vi "_LogFirmwareEvents.vi"(0 "Event":string="117:52:56, Lost Communication - Check Ethernet Connection.\n117:52:56, Going to Lost Communication state.\n117:52:56, Instr State transitioned from Ready to Lost Communication; FPGA Running = FALSE; Run Mode = 1; Loop = 431971.\n117:52:56, Heater Power Supply Error; Instr State = Lost Communication.\n117:52:56, PC Communication Established\n117:55:43, Start Run: Instr State = Lost Communication; FPGA Running = FALSE;  Time Out = FALSE.\n117:55:44, Analyzer is Ready\n117:55:52, Start Run: Instr State = Ready; FPGA Running = FALSE;  Time Out = FALSE.\n117:55:56, Heater Power Supply Error; Instr State = Ready.") -> ()   [LabVIEW 2015]
doc: "This vi maintains a datalog file for plate positions in motor steps.\nEach datalog record consists of the following data members:\nData/time in secs from 12am 1/1/1904.\nHorizontal motor steps\nVertical motor steps\nAll numbers are stored as 8-byte doubles."
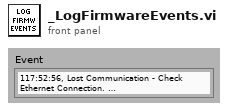
[diagram p1: front panel]
types:
  T1 = enum16{"open", "replace", "create", "open or create", "replace or create", "replace or create with confirmation"}
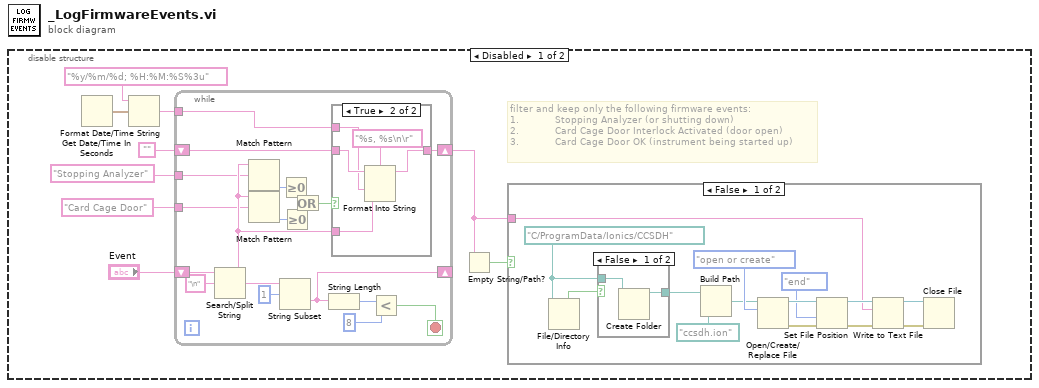
[diagram p0: block diagram]
diagram:
  n1 = disable-structure shown="Disabled" {
    frame Disabled {
      # "filter and keep only the following firmware events:\n1.            Stopping Analyzer (or shutting down)\n2.            Card Cage Door Interlock Activated (door open)\n3.            Card Cage Door OK (instrument being started up)"
      n2 = Get Date/Time In Seconds() -> (seconds since 1Jan1904=w6:timestamp)
      n3 = Format Date/Time String(time format string (%c)="%y/%m/%d; %H:%M:%S%3u", seconds (now)=w6) -> (date/time string=w4:string)  [unwired: 1 out]
      n4 = while {
        shift-right: [w19] -> w3
        shift-left: "" -> [w20]
        tunnel: w4 -> [w18]
        shift-right: [w24] -> _
        shift-left: "Event" -> [w28]
        tunnel: "Stopping Analyzer" -> [w16]
        tunnel: "Card Cage Door" -> [w15]
        stop <- w22 stop-if-true
        n5 = Search/Split String(string=w28, search string/char (-)="\n") -> (substring before match=w17:string, match + rest of string=w26:string)  [unwired: 1 in, 1 out]
        n6 = Match Pattern(string=w17, regular expression=w16) -> (offset past match=w14:i32)  [unwired: 1 in, 3 out]
        n7 = Match Pattern(string=w17, regular expression=w15) -> (offset past match=w13:i32)  [unwired: 1 in, 3 out]
        n8 = String Subset(string=w26, offset (0)=1) -> (substring=w24:string)  [unwired: 1 in]
        n9 = Greater Or Equal To 0?(x=w14) -> (x >= 0?=w11:bool)
        n10 = Greater Or Equal To 0?(x=w13) -> (x >= 0?=w10:bool)
        n11 = Or(x=w11, y=w10) -> (x .or. y?=w12:bool)
        n12 = String Length(string=w24) -> (length=w23:i32)
        n13 = case shown="True" w12 {
          tunnel: w20 -> [w29 w33]
          tunnel: [w29 w30] -> w19
          tunnel: w18 -> [_ w32]
          tunnel: w17 -> [_ w31]
          frame False {
          }
          frame True {
            n14 = Format Into String(format string="%s, %s\n\r" ("Format String"), initial string=w33, w32, w31) -> (resulting string=w30:string)  [unwired: 1 in, 1 out]
          }
        }
        n15 = Less?(x=w23, y=8) -> (x < y?=w22:bool)
      }
      n16 = Empty String/Path?(string/path=w3) -> (empty?=w9:bool)
      n17 = case shown="False" w9 {
        tunnel: w3 -> [w35 _]
        frame False {
          w47 = path "C:/ProgramData/Ionics/CCSDH" ("path")
          n18 = File/Directory Info(path=w47) -> (directory=w48:bool)  [unwired: 1 in, 6 out]
          n19 = case shown="False" w48 {
            tunnel: w47 -> [w50 w51]
            tunnel: [w49 w51] -> w46
            frame False {
              n20 = Create Folder(path (use dialog)=w50) -> (created path=w49:path)  [unwired: 2 in, 2 out]
            }
            frame True {
            }
          }
          n21 = Build Path(base path=w46, name or relative path=path "ccsdh.ion" ("configuration file path")) -> (appended path=w43:path)
          n22 = Open/Create/Replace File(file path (use dialog)=w43, operation (0:open)=T1."open or create") -> (refnum out=w40:refnum<file>, error out=w38:errorcluster)  [unwired: 4 in, 1 out]
          n23 = Set File Position(refnum=w40, from (0:start)=enum16{"start", "end", "current"}."end", error in=w38) -> (refnum out=w39:refnum<file>, error out=w37:errorcluster)  [unwired: 1 in]
          n24 = Write to Text File(file (use dialog)=w39, text=w35, error in=w37) -> (refnum out=w42:refnum<file>, error out=w41:errorcluster)  [unwired: 1 in, 1 out]
          n25 = Close File(refnum=w42, error in=w41) -> ()  [unwired: 2 out]
        }
        frame True {
        }
      }
    }
    frame Enabled {
    }
  }
